vi "From Paths.vi"(0 "Paths":path[](array[path])) -> (2 "Array":refnum<class "Array.lvclass">)   [LabVIEW 2018, in "Toolkit.lvlib" / "Types.lvlib" / "Array.lvclass"]
uses:
  Array.lvclass
  Array.lvclass/Array.ctl
  Path/Path.lvclass
  D:/Users/cfield/Code/Field R&D Services/Mustache/LabVIEW/trunk/src/Toolkit/Data/Abstract/Abstract.lvclass
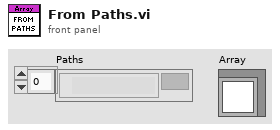
[diagram p1: front panel]
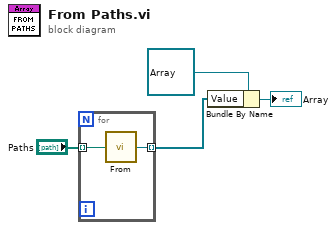
[diagram p0: block diagram]
diagram:
  n1 = for {
    tunnel: "Paths" -> [w6] mode=indexing
    tunnel: [w5] -> w2 mode=indexing
    n2 = call "From.vi"("Value"=w6) -> ("Path"=w5:refnum<class "Path.lvclass">)
  }
  n3 = Bundle By Name(cluster=refnum<class "Array.lvclass"> refnum ("Toolkit.lvlib:Data.lvlib:Array.lvclass"), "Value"=w2) -> (→"Array":refnum<class "Array.lvclass">)
